vi "OpenAnotherVI.vi"(8 "error in (no error)":errorcluster, 9 "State":T1(ring), 10 "vi path 2":path, 11 "vi path":path) -> (0 "error out":errorcluster)   [LabVIEW 2017]
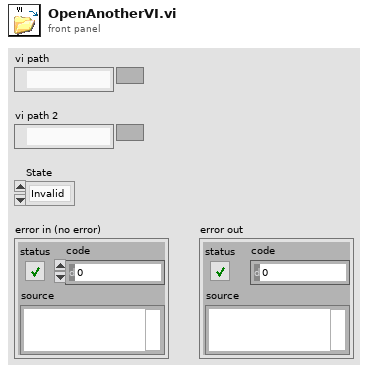
[diagram p1: front panel]
types:
  T1 = enum32{"Invalid", "Standard", "Closed", "Hidden", "Minimized", "Maximized"}
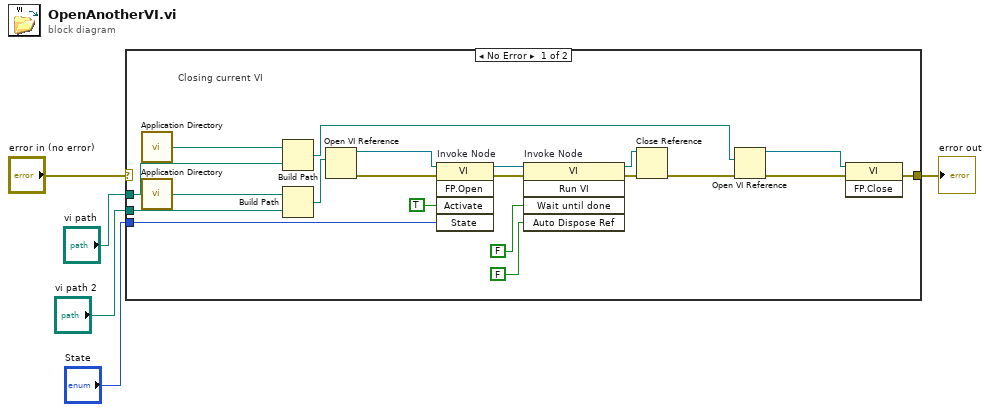
[diagram p0: block diagram]
diagram:
  n1 = case shown="No Error" "error in (no error)" {
    selector: "error in (no error)" -> [_ w26]
    tunnel: [w10 w26] -> w4
    tunnel: "vi path 2" -> [w24 _]
    tunnel: "State" -> [w16 _]
    tunnel: "vi path" -> [w8 _]
    frame No Error {
      # "Closing current VI"
      n2 = call <vilib>:"Application Directory.vi"() -> ("Application Directory"=w9:path)
      n3 = call <vilib>:"Application Directory.vi"() -> ("Application Directory"=w23:path)
      n4 = Build Path(base path=w9, name or relative path=w8) -> (appended path=w6:path)
      n5 = Build Path(base path=w23, name or relative path=w24) -> (appended path=w25:path)
      n6 = Open VI Reference(vi path=w25) -> (vi reference=w13:refnum<vi>, error out=w14:errorcluster)  [unwired: 1 in, 4 out]
      n7 = invoke on="Invoke Node" class="VI" method="FP.Open"(reference=w13, error in=w14, "Activate"=TRUE ("Activate?"), "State"=w16) -> (reference out=w17:refnum<vi>, error out=w18:errorcluster)  [unwired: 1 in, 3 out]
      n8 = invoke on="Invoke Node" class="VI" method="Run VI"(reference=w17, error in=w18, "Wait until done"=FALSE ("Wait Until Done"), "Auto Dispose Ref"=FALSE ("Auto Dispose Reference")) -> (reference out=w21:refnum<vi>, error out=w22:errorcluster)  [unwired: 1 in, 3 out]
      n9 = Close Reference(reference=w21, error in (no error)=w22) -> (error out=w7:errorcluster)
      n10 = Open VI Reference(vi path=w6, error in (no error)=w7) -> (vi reference=w12:refnum<vi>, error out=w11:errorcluster)  [unwired: 4 out]
      n11 = invoke class="VI" method="FP.Close"(reference=w12, error in=w11) -> (error out=w10:errorcluster)  [unwired: 1 in, 2 out]
    }
    frame Error {
    }
  }
  "error out" <- w4
